vi "Write Clock Rate (Hz).vi"(8 "error in (no error)":errorcluster, 10 "Clock Rate (Hz)":dbl=500000.0, 11 "navX - SPI in":refnum<class "navX - SPI.lvclass">) -> (0 "error out":errorcluster, 3 "navX - SPI out":refnum<class "navX - SPI.lvclass">)   [LabVIEW 2015, in "navX Library v3.lvlib" / "navX - SPI.lvclass"]
uses:
  navX - SPI.lvclass
  navX - SPI.lvclass/navX - SPI.ctl
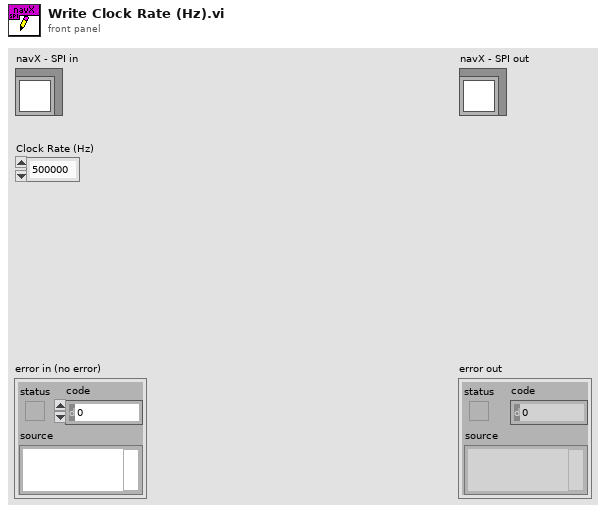
[diagram p1: front panel]
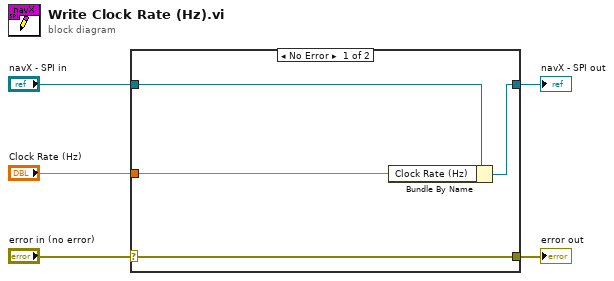
[diagram p0: block diagram]
diagram:
  n1 = case shown="No Error" "error in (no error)" {
    selector: "error in (no error)" -> [w9 w10]
    tunnel: [w9 w10] -> w4
    tunnel: [w7 w11] -> w2
    tunnel: "navX - SPI in" -> [w8 w11]
    tunnel: "Clock Rate (Hz)" -> [w6 _]
    frame No Error {
      n2 = Bundle By Name(cluster=w8, "Clock Rate (Hz)"=w6) -> (w7:refnum<class "navX - SPI.lvclass">)
    }
    frame Error {
    }
  }
  "error out" <- w4
  "navX - SPI out" <- w2
